vi "Write Configuration Data.vi"(8 "error in (no error)":errorcluster, 10 "Configuration Settings":T1={"Offset"=0.0, "Signal Type"=enum."Sine Wave", "Frequency"=10.0, "Amplitude"=1.0, "Phase"=0.0, "Noise Amplitude"=1.0} {"Noise Amplitude" format="%.2p"; "Phase" format="%.2p"; "Amplitude" format="%0.2p"; "Frequency" format="%0.2p"; "Offset" format="%0.2p"}, 11 "Path":path) -> (0 "error out":errorcluster)   [LabVIEW 2020]
uses:
  Controls/Configuration Settings.ctl
  <vilib>/Utility/config.llb/Write Key (Double).vi
  <vilib>/Utility/config.llb/Write Key (U32).vi
  <vilib>/Utility/config.llb/NI_LVConfig.lvlib
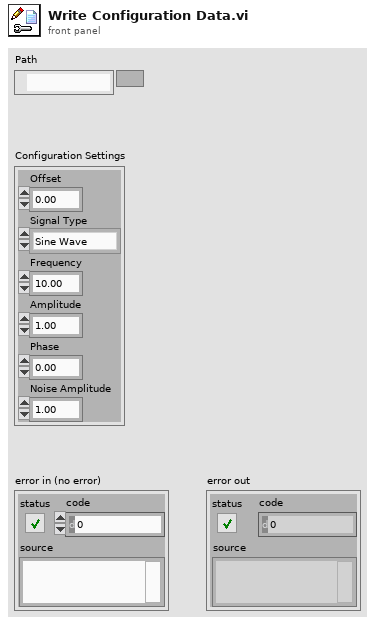
[diagram p1: front panel]
types:
  T1 = typedef "Configuration Settings.ctl" = cluster{"Offset":dbl, "Signal Type":enum16{"Sine Wave", "Triangle Wave", "Square Wave", "Sawtooth Wave"}, "Frequency":dbl, "Amplitude":dbl, "Phase":dbl, "Noise Amplitude":dbl}
  T2 = enum16{"Sine Wave", "Triangle Wave", "Square Wave", "Sawtooth Wave"}
  T3 = typedef "NI_LVConfig.lvlib/Config Data RefNum.ctl" = refnum<k1>
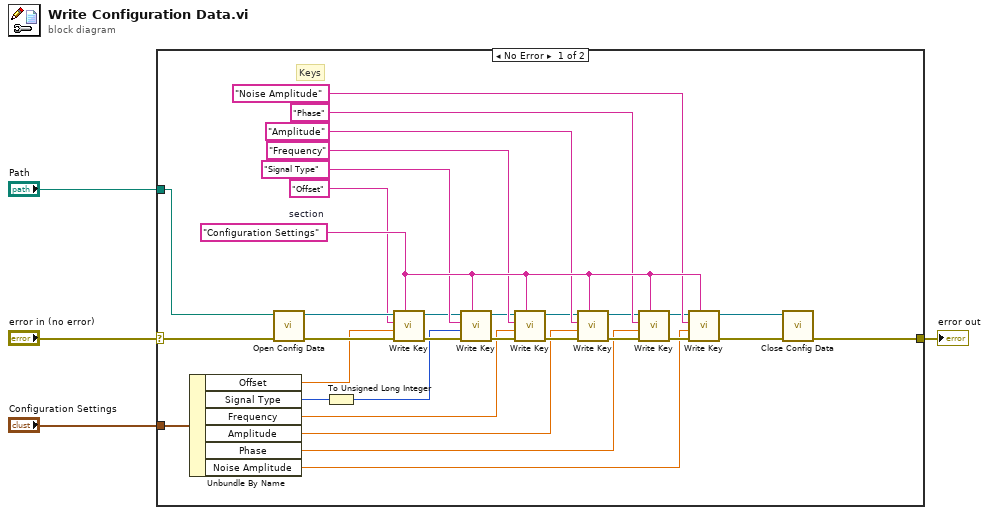
[diagram p0: block diagram]
diagram:
  n1 = case shown="No Error" "error in (no error)" {
    selector: "error in (no error)" -> [w34 w37]
    tunnel: [w12 w37] -> w3
    tunnel: "Configuration Settings" -> [w36 _]
    tunnel: "Path" -> [w35 _]
    frame No Error {
      w32 = "Configuration Settings"  # section
      # "Keys"
      n2 = Unbundle By Name(w36) -> ("Offset"=w11:dbl, "Signal Type"=w10:T2, "Frequency"=w9:dbl, "Amplitude"=w8:dbl, "Phase"=w7:dbl, "Noise Amplitude"=w6:dbl)
      n3 = call <vilib>:"Open Config Data.vi"("error in (no error)"=w34, "configuration file path"=w35) -> ("error out"=w13:errorcluster, "refnum"=w33:T3)  [unwired: 7 in, 1 out]
      n4 = To Unsigned Long Integer(number=w10) -> (unsigned 32bit integer=w5:u32)
      n5 = call-poly <vilib>:"Write Key.vi"("section"=w32, "error in (no error)"=w13, "value"=w11, "key"="Offset" ("Key"), "refnum"=w33) -> ("error out"=w14:errorcluster, "refnum out"=w25:T3)  [unwired: 4 in, 1 out]
      n6 = call-poly <vilib>:"Write Key.vi"("section"=w32, "error in (no error)"=w14, "value"=w5, "key"="Signal Type" ("Key"), "refnum"=w25) -> ("error out"=w15:errorcluster, "refnum out"=w24:T3)  [unwired: 4 in, 1 out]
      n7 = call-poly <vilib>:"Write Key.vi"("section"=w32, "error in (no error)"=w15, "value"=w9, "key"="Frequency" ("Key"), "refnum"=w24) -> ("error out"=w16:errorcluster, "refnum out"=w23:T3)  [unwired: 4 in, 1 out]
      n8 = call-poly <vilib>:"Write Key.vi"("section"=w32, "error in (no error)"=w16, "value"=w8, "key"="Amplitude" ("Key"), "refnum"=w23) -> ("error out"=w17:errorcluster, "refnum out"=w22:T3)  [unwired: 4 in, 1 out]
      n9 = call-poly <vilib>:"Write Key.vi"("section"=w32, "error in (no error)"=w17, "value"=w7, "key"="Phase" ("Key"), "refnum"=w22) -> ("error out"=w18:errorcluster, "refnum out"=w21:T3)  [unwired: 4 in, 1 out]
      n10 = call-poly <vilib>:"Write Key.vi"("section"=w32, "error in (no error)"=w18, "value"=w6, "key"="Noise Amplitude" ("Key"), "refnum"=w21) -> ("error out"=w19:errorcluster, "refnum out"=w20:T3)  [unwired: 4 in, 1 out]
      n11 = call <vilib>:"Close Config Data.vi"("error in (no error)"=w19, "refnum"=w20) -> ("error out"=w12:errorcluster)  [unwired: 8 in, 1 out]
    }
    frame Error {
    }
  }
  "error out" <- w3
